vi "read_u8 array.vi"(8 "error in (no error)":errorcluster caption="에러 입력(에러 없음)", 9 "size to read":u32=1, 10 "start address":u32, 11 "I2C 입력":refnum<class "I2C.lvclass">) -> (0 "error out":errorcluster caption="에러 출력", 1 "data out":u8[](array[numeric]), 2 "log_multiple line":string[](array[string]), 3 "I2C 출력":refnum<class "I2C.lvclass">, 4 "log_single line":string[](array[string]))   [LabVIEW 2020, in "I2C.lvclass"]
uses:
  I2C.lvclass
  I2C.lvclass/I2C.ctl
  SubVIs/Serial/Controls/(Ctrl)Serial_Write Read Option.ctl
  Controls/(Ctrl)log & script_rw enum.ctl
  Accessors/Read data byte.vi
  Accessors/Read address byte.vi
  Accessors/Read clock rate.vi
  Accessors/Read slave address.vi
  Variables/(Var)System Variables.vi
  SubVIs/Serial/Instance VIs/(SubVI)Serial_Write-Read.vi
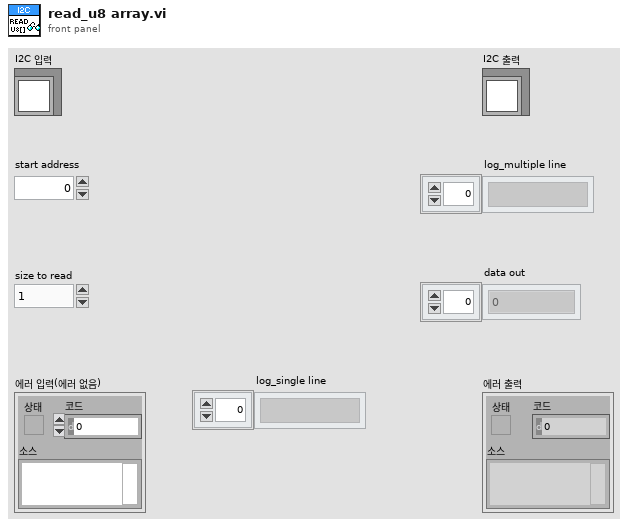
[diagram p1: front panel]
types:
  T1 = typedef "I2C.lvclass/(Ctrl)log & script_rw enum.ctl" = enum16{"Read", "Write"}
  T2 = typedef "(Ctrl)Serial_Write Read Option.ctl" = cluster{"Echo Request":bool, "Header Verification":bool, "Checksum Verification":bool, "User Code Verifiaction":bool}
  T3 = typedef "IC I2C Clock Rate.ctl" = enum8{"50khz", "100khz", "400khz", "1Mhz", "1.2Mhz"}
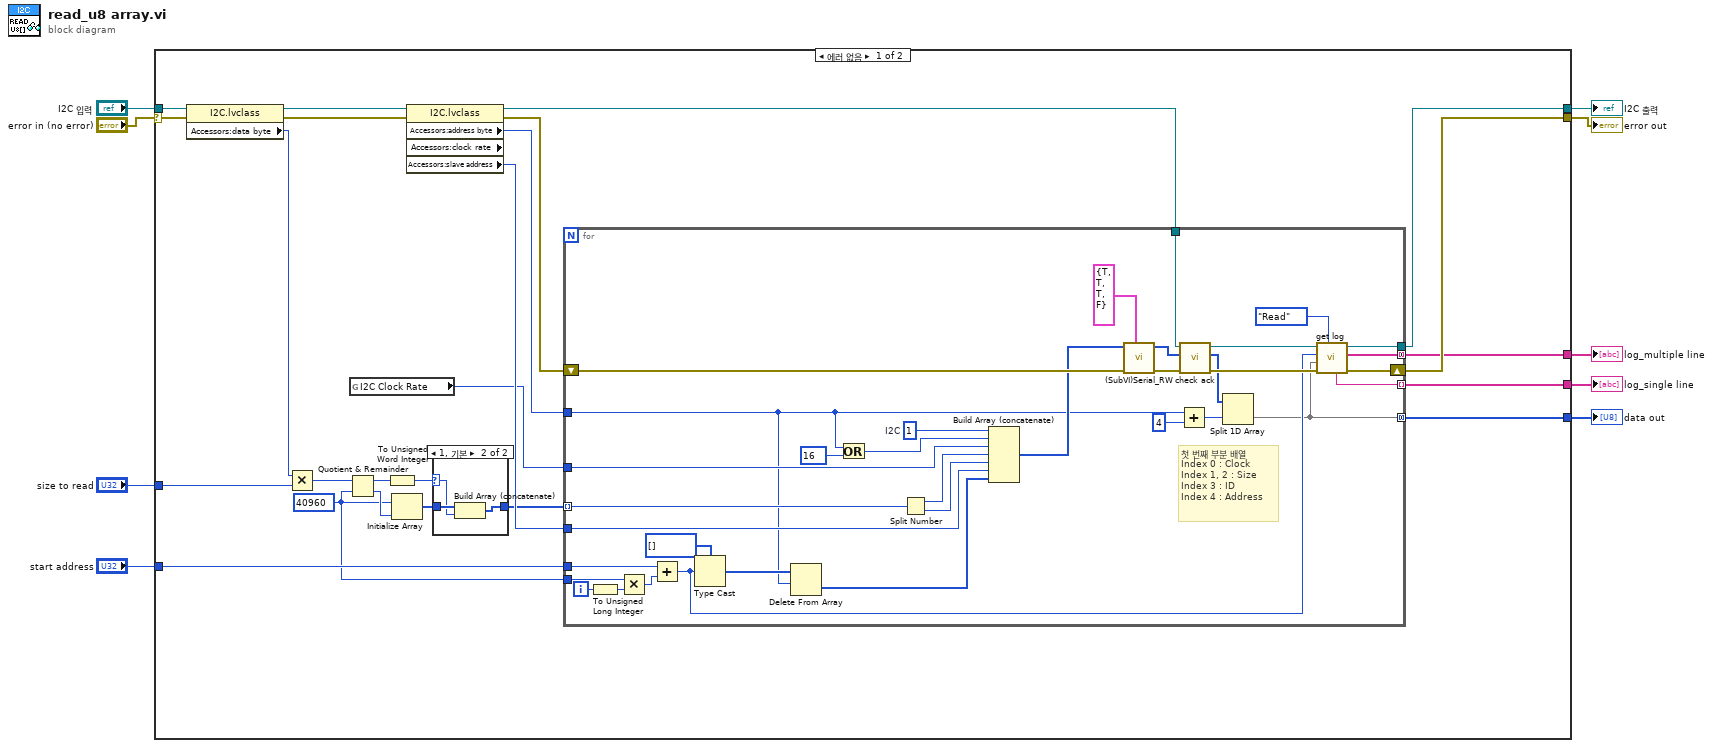
[diagram p0: block diagram]
diagram:
  n1 = case shown="에러 없음" "error in (no error)" {
    selector: "error in (no error)" -> [w33 w74]
    tunnel: [w30 w74] -> w8
    tunnel: [w18 w73] -> w6
    tunnel: "I2C 입력" -> [w16 w73]
    tunnel: "start address" -> [w32 _]
    tunnel: [w27 _] -> w4
    tunnel: "size to read" -> [w23 _]
    tunnel: [w12 _] -> w2
    tunnel: [w11 _] -> w1
    frame No Error {
      w20 = u16 40960 ("y")
      n2 = property class="I2C.lvclass"(reference=w16, error in=w33) -> (reference out=w15:refnum<class "I2C.lvclass">, error out=w17:errorcluster, "Accessors:data byte"=w13:u8)
      n3 = Multiply(x=w13, y=w23) -> (x*y=w14:u32)
      n4 = Quotient & Remainder(x=w14, y=w20) -> (x-y*floor(x/y)=w26:u32, floor(x/y)=w24:u32)
      n5 = global read "(Var)System Variables.vi" "I2C Clock Rate"() -> (w10:T3)
      n6 = To Unsigned Word Integer(number=w26) -> (unsigned 16bit integer=w21:u16)
      n7 = Initialize Array(w20, w24) -> (w25:u16[])
      n8 = property class="I2C.lvclass" props=["Accessors:address byte", "Accessors:clock rate", "Accessors:slave address"](reference=w15, error in=w17) -> (reference out=w19:refnum<class "I2C.lvclass">, error out=w31:errorcluster, "Accessors:address byte"=w28:u8, "Accessors:slave address"=w29:u8)  [unwired: 1 out]
      n9 = case shown="1, 기본" w21 {
        selector: w21 -> [_ w35]
        tunnel: w25 -> [w34 w37]
        tunnel: [w34 w36] -> w22
        frame 0 {
        }
        frame 1, Default {
          n10 = Build Array (concatenate)(w37, w35) -> (w36:u16[])
        }
      }
      n11 = for {
        tunnel: w32 -> [w63]
        shift-right: [w45] -> w30
        shift-left: w31 -> [w72]
        tunnel: [w39] -> w27 mode=concatenating
        tunnel: w29 -> [w61]
        tunnel: w10 -> [w48]
        tunnel: w28 -> [w46]
        tunnel: w22 -> [w58] mode=indexing
        tunnel: w20 -> [w56]
        tunnel: w19 -> [w54]
        tunnel: [w43] -> w18
        tunnel: [w42] -> w12 mode=concatenating
        tunnel: [w38] -> w11 mode=indexing
        i -> [w62]
        w71 = u8 1  # I2C
        # "첫 번째 부분 배열\nIndex 0 : Clock\nIndex 1, 2 : Size\nIndex 3 : ID\nIndex 4 : Address"
        n12 = To Unsigned Long Integer(number=w62) -> (unsigned 32bit integer=w55:u32)
        n13 = Multiply(x=w56, y=w55) -> (x*y=w57:u32)
        n14 = Add(x=w63, y=w57) -> (x+y=w40:u32)
        n15 = Type Cast(type=u8[] [] ("타입"), x=w40) -> (*(type *) &x=w47:u8[])
        n16 = Delete From Array(array=w47, length=w46) -> (deleted portion=w59:u8[])  [unwired: 1 in, 1 out]
        n17 = Or(x=w46, y=u8 16) -> (x .or. y?=w50:u8)
        n18 = Split Number(x=w58) -> (hi(x)=w70:u8, lo(x)=w69:u8)
        n19 = Build Array (concatenate)(w71, w50, w48, w70, w69, w61, w59) -> (w64:u8[])
        n20 = call-poly "(SubVI)Serial_RW.vi"("Option"=T2 {"Echo Request"=TRUE, "Header Verification"=TRUE, "Checksum Verification"=TRUE, "User Code Verifiaction"=FALSE}, "error in (no error)"=w72, "Data to Write"=w64) -> ("error out"=w67:errorcluster, "Read Data"=w66:u8[])  [unwired: 6 in, 1 out]
        n21 = Add(x=w46, y=4 ("인덱스")) -> (x+y=w51:i32)
        n22 = call-dynamic "check ack.vi"("error in (no error)"=w67, "Read Data"=w66, "I2C 입력"=w54) -> ("error out"=w68:errorcluster, "Read Data Out"=w52:u8[], "I2C 출력"=w44:refnum<class "I2C.lvclass">)  [unwired: 6 in]
        n23 = Split 1D Array(array=w52, index=w51) -> (second subarray=w39:u8[])  [unwired: 1 out]
        n24 = call-dynamic "get log.vi"("rw"=(Ctrl)log_&_script_rw_enum."Read", "error in (no error)"=w68, "data"=w39, "start addr"=w40, "I2C 입력"=w44) -> ("error out"=w45:errorcluster, "log_multiple line"=w42:string[], "I2C 출력"=w43:refnum<class "I2C.lvclass">, "log_single line"=w38:string)  [unwired: 3 in]
      }
    }
    frame Error {
    }
  }
  "error out" <- w8
  "I2C 출력" <- w6
  "data out" <- w4
  "log_multiple line" <- w2
  "log_single line" <- w1
